vi "comunicacao.vi"() -> ()   [LabVIEW 2019]
panel:
  in  "comunicacao":bool
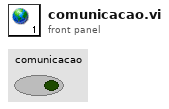
[diagram p1: front panel]
diagram:
